vi "Calibration Insert Parameters.vi"(8 "error in (no error)":errorcluster, 11 "VariableValue":string) -> (0 "error out":errorcluster, 3 "Insert DB String":string)   [LabVIEW 2017, in "SQLite.lvclass"]
doc: "insert the parameters into Parameter Tabel in Calibration DB.\n2016-03-17 12:52:18\n蒋松\nsina: @sushu1051"
uses:
  SQLite.lvclass
  SQLiteFileName.ctl
  TabelFullName.ctl
  <userlib>/LabSQL/LabSQL.lvlib
  <userlib>/sushu/sushu.lvlib
panel:
  out "Insert DB String 2":string
  out "Select SQL CMD":string
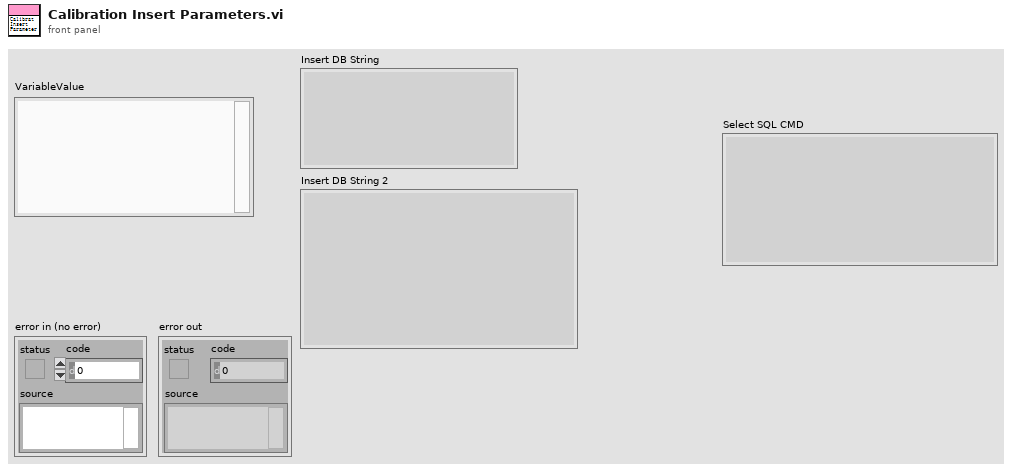
[diagram p1: front panel]
types:
  T1 = enum16{"Other", "SQL2008", "SQLite", "Access", "MySQL"}
  T2 = typedef "SQLite.lvclass/TabelFullName.ctl" = string
  T3 = typedef "SQLite.lvclass/SQLiteFileName.ctl" = string
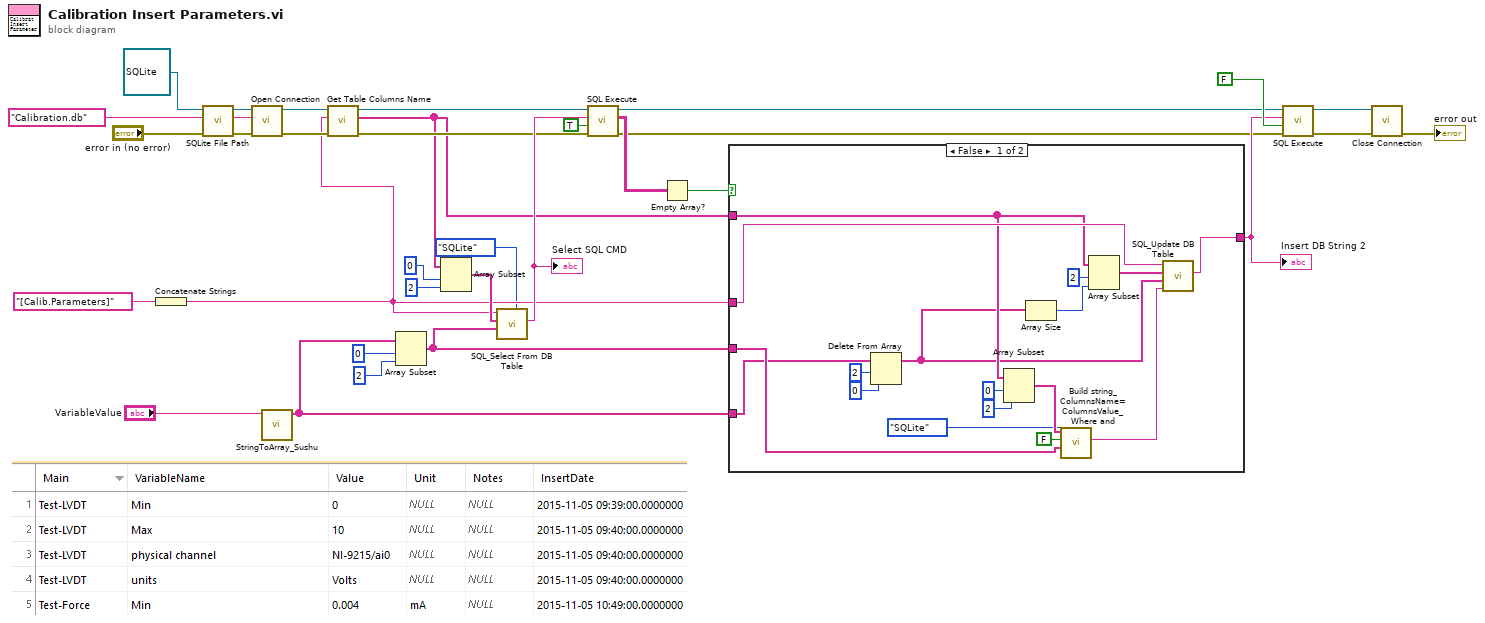
[diagram p0: block diagram]
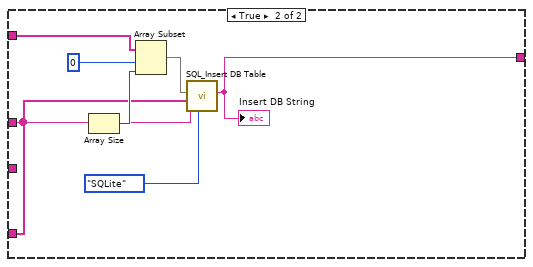
[diagram p2: hidden frame]
diagram:
  n1 = Concatenate Strings(T2 "[Calib.Parameters]" ("TabelFullName")) -> (w8:string)
  n2 = call "SQLite File Path.vi"("error in (no error)"="error in (no error)", "SQLiteFileName"=T3 "Calibration.db", "SQLite in"=refnum<class "SQLite.lvclass"> refnum ("SQLite.lvclass")) -> ("error out"=w32:errorcluster, "string"=w24:string, "SQLite out"=w26:refnum<class "SQLite.lvclass">)  [unwired: 6 in]
  n3 = call-dynamic "Open Connection.vi"("error in (no error)"=w32, "ConnectionString"=w24, "HostDB in"=w26) -> ("error out"=w23:errorcluster, "HostDB out"=w22:refnum<class "SQLite.lvclass">)  [unwired: 7 in]
  n4 = call <userlib>:"StringToArray_Sushu.vi"("State Queue"="VariableValue") -> ("Array"=w5:string[])  [unwired: 8 in, 2 out]
  n5 = call-dynamic "Get Table Columns Name.vi"("error in (no error)"=w23, "TableName"=w8, "HostDB in"=w22) -> ("error out"=w11:errorcluster, "ColunmsList"=w9:string[], "HostDB out"=w13:refnum<class "SQLite.lvclass">)  [unwired: 4 in, 2 out]
  n6 = Array Subset(array=w5, index=0, length=2) -> (w3:string[])
  n7 = Array Subset(array=w9, index=0, length=2) -> (w17:string[])
  n8 = call <userlib>:"SQL_Select From DB Table.vi"("DB Type"=T1."SQLite", "ColumnsValue"=w3, "ColumnsNameList"=w17, "TableName"=w8) -> ("Select SQL CMD"=w15:string)  [unwired: 7 in]
  "Select SQL CMD" <- w15
  n9 = call-dynamic "SQL Execute.vi"("error in (no error)"=w11, "Return Data (T)"=TRUE, "Command Text"=w15, "HostDB in"=w13) -> ("error out"=w10:errorcluster, "Table Control"=w14:string[][], "HostDB out"=w12:refnum<class "SQLite.lvclass">)  [unwired: 3 in, 2 out]
  n10 = Empty Array?(array=w14) -> (empty?=w4:bool)
  n11 = case shown="False" w4 {
    tunnel: [w35 w55] -> w19
    tunnel: w9 -> [w41 w53]
    tunnel: w8 -> [w42 w52]
    tunnel: w5 -> [w39 w51]
    tunnel: w3 -> [w40 _]
    frame False {
      n12 = Delete From Array(array=w39, length=2, index=0) -> (array with subset deleted=w36:string[])  [unwired: 1 out]
      n13 = Array Subset(array=w41, index=0, length=2) -> (w48:string[])
      n14 = Array Size(array=w36) -> (size(s)=w45:i32)
      n15 = call <userlib>:"Build string_ColumnsName=ColumnsValue_Where and.vi"("DB Type"=T1."SQLite", "ColumnsValue"=w40, "Check ASCII?"=FALSE, "ColumnsNameList"=w48) -> ("ColumnName='ColumnValue'"=w50:string)  [unwired: 7 in]
      n16 = Array Subset(array=w41, index=2, length=w45) -> (w43:string[])
      n17 = call <userlib>:"SQL_Update DB Table.vi"("where name='value'"=w50, "ColumnsValue"=w36, "ColumnsNameList"=w43, "TableName"=w42) -> ("Update CMD"=w35:string)  [unwired: 7 in]
    }
    frame True {
      n18 = Array Size(array=w51) -> (size(s)=w57:i32)
      n19 = Array Subset(array=w53, index=0, length=w57) -> (w56:string[])
      n20 = call <userlib>:"SQL_Insert DB Table.vi"("DB Type"=enum16{"Other", "SQL2008", "SQLite"}."SQLite", "ColumnsValue"=w51, "ColumnsName"=w56, "Table Name"=w52) -> ("Insert DB String"=w55:string)  [unwired: 7 in]
      "Insert DB String" <- w55
    }
  }
  "Insert DB String 2" <- w19
  n21 = call-dynamic "SQL Execute.vi"("error in (no error)"=w10, "Return Data (T)"=FALSE, "Command Text"=w19, "HostDB in"=w12) -> ("error out"=w31:errorcluster, "HostDB out"=w30:refnum<class "SQLite.lvclass">)  [unwired: 3 in, 3 out]
  n22 = call-dynamic "Close Connection.vi"("error in (no error)"=w31, "HostDB in"=w30) -> ("error out"=→"error out":errorcluster)  [unwired: 8 in, 1 out]
